vi "PH_HamamatsuCamera.Setting Packer.vi"(0 "i ref in":refnum<vi>, 5 "error in (no error)":errorcluster) -> (14 "i ref out":refnum<vi>, 18 "Cam Settings":T1={"Cam ID"="N/A", "Gain"=nan, "Brightness"=nan, "Shutter"=nan, "Mode"=-1}, 19 "error out":errorcluster)   [LabVIEW 2014, in "PH_HamamatsuCamera.lvlib"]
doc: "This VI gets the cam settings from own attributes, labels them, and packs them to a string array."
uses:
  PH_HamamatsuCamera.lvlib
  PH_Cam_BaseClass/PH_Cam_BaseClass.Settings.ctl
  PH_Cam_BaseClass/PH_Cam_BaseClass.lvlib
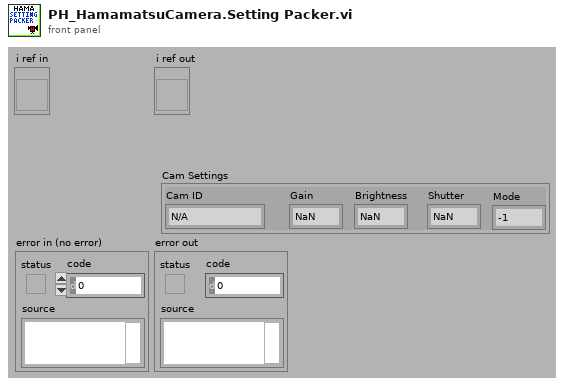
[diagram p1: front panel]
types:
  T1 = typedef "PH_Cam_BaseClass.lvlib/PH_Cam_BaseClass.Settings.ctl" = cluster{"Cam ID":string, "Gain":dbl, "Brightness":dbl, "Shutter":dbl, "Mode":i32}
  T2 = typedef "PH_HamamatsuCamera.lvlib/PH_HamamatsuCamera.i attribute.ctl" = cluster{"Gui Refs":cluster{"Camera Details":refnum<vi>, "ROI":refnum<vi>, "Set ROI to Maximum":refnum<vi>, "Trigger Parameters":refnum<vi>, "Brightness":refnum<vi>, "Shutter":refnum<vi>, "Gain":refnum<vi>, "Trigger Timeout":refnum<vi>, "Trigger Polarity":refnum<vi>, "Trigger Mode":refnum<vi>, "Parameters":refnum<vi>, "Set Cam Parameter":refnum<vi>, "Parameter to set":refnum<vi>, "Value to set":refnum<vi>}, "Cam":cluster{"Handle":i32, "Details":cluster{"Model":string, "Camera ID":string, "Firmware":string}, "Buffer Info":cluster{"height":u32, "width":u32, "datatype":u32}}, "H Offset":cluster{"Value":i32, "Minimum":i32, "Maximum":i32, "Increment":i32}, "V Offset":cluster{"Value":i32, "Minimum":i32, "Maximum":i32, "Increment":i32}, "H Width":cluster{"Value":i32, "Minimum":i32, "Maximum":i32, "Increment":i32}, "V Width":cluster{"Value":i32, "Minimum":i32, "Maximum":i32, "Increment":i32}, "Trigger Parameters":T3, "Trigger Timeout":u32, "Parameters":T4[], "Indicees Cam Parameters":cluster{"Brightness":i32, "Shutter":i32, "Gain":i32}, "Wanted Values":cluster{"Trigger Settings":T3[], "ROI":T5[], "Parameter":cluster{"Name":string, "Value":dbl}[]}}
  T3 = typedef "PH_HamamatsuCamera.lvlib/PH_HamamatsuCamera.Trigger Parameter.ctl" = cluster{"Mode":u32, "Polarity":u32, "Times":u32, "Delay":dbl}
  T4 = typedef "PH_HamamatsuCamera.lvlib/PH_HamamatsuCamera.Parameter Set.ctl" = cluster{"Parameter":string, "Value":dbl, "Writable":bool, "Range":cluster{"min":dbl, "max":dbl, "step":dbl}, "Default":dbl, "Value Names":cluster{"Name":string, "Value":dbl}[], "Text Values":bool}
  T5 = typedef "PH_HamamatsuCamera.lvlib/PH_HamamatsuCamera.ROI.ctl" = cluster{"Horizontal Offset":i32, "Vertical Offset":i32, "Horizontal Width":i32, "Vertical Width":i32}
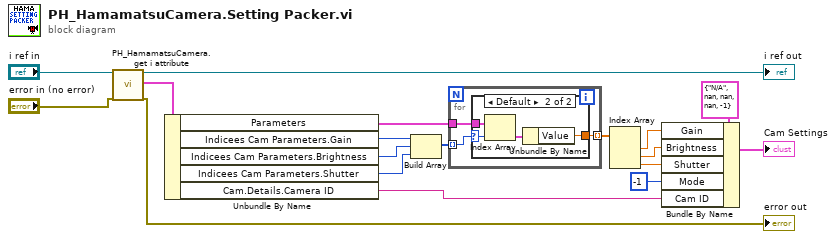
[diagram p0: block diagram]
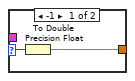
[diagram p2: hidden frame]
diagram:
  n1 = call "PH_HamamatsuCamera.get i attribute.vi"("i ref in"="i ref in", "error in (no error)"="error in (no error)") -> ("i ref out"=→"i ref out":refnum<vi>, "i attribute"=w18:T2, "error out"=→"error out":errorcluster)  [unwired: 15 in]
  n2 = Unbundle By Name(w18) -> ("Parameters"=w10:T4[], "Indicees Cam Parameters.Gain"=w14:i32, "Indicees Cam Parameters.Brightness"=w13:i32, "Indicees Cam Parameters.Shutter"=w12:i32, "Cam.Details.Camera ID"=w2:string)
  n3 = Build Array(w14, w13, w12) -> (w11:i32[])
  n4 = for {
    tunnel: w11 -> [w19] mode=indexing
    tunnel: w10 -> [w21]
    tunnel: [w20] -> w7 mode=indexing
    n5 = case shown="Default" w19 {
      selector: w19 -> [w23 w25]
      tunnel: w21 -> [_ w27]
      tunnel: [w22 w24] -> w20
      frame -1 {
        n6 = To Double Precision Float(number=w23) -> (double precision float=w22:dbl)
      }
      frame Default {
        n7 = Index Array(array=w27, index=w25) -> (element=w26:T4)
        n8 = Unbundle By Name(w26) -> ("Value"=w24:dbl)
      }
    }
  }
  n9 = Index Array(array=w7) -> (element #1=w6:dbl, element #2=w4:dbl, element #3=w5:dbl)  [unwired: 3 in]
  n10 = Bundle By Name(cluster=T1 {"Cam ID"="N/A", "Gain"=nan, "Brightness"=nan, "Shutter"=nan, "Mode"=-1} ("Cam Settings"), "Gain"=w6, "Brightness"=w4, "Shutter"=w5, "Mode"=-1 ("Video Mode"), "Cam ID"=w2) -> (→"Cam Settings":T1)
